vi "SRQ Event Handling.vi"() -> ()   [LabVIEW 2020]
doc: "This example detects and responds to a service request (SRQ) event. It shows a generic method to generate and handle an SRQ event. But each instrument that supports SRQ event assertion will use a different set of commands than what is shown in this example. You will need to refer to the programmer reference manual for your particular instrument to determine the correct set of commands."
uses:
  <vilib>/Instr/_visa.llb/Select Event Type.ctl
panel:
  in  "Command":string="*ESE 0x01; *SRE 0x30; SOUR:FUNC SIN;*OPC;SENS:DATA?"
  out "status byte":u16
  out "Raw Data":string
  in  "VISA GPIB Resource":refnum<visa-resource-name>="GPIB0::3::INSTR"
  # "Overview: Detects and responds to a service request (SRQ) event sent by a GPIB device.\nRequirements: NI-488.2 and NI-VISA Drivers\nInstructions:\n1. Ensure the resource specified in the VISA GPIB Resource control is properly configured in Measurement & Automation Explorer.\n2. Run the VI.\n3. If your instrument recognizes the Command specified below, it should return a response in the Raw Data."
  # "Service Request (SRQ) events are sent by GPIB devices to the controller to request service. The Command string in this example which instructs the instrument to generate an SRQ may need to be modified for your specific instrument."
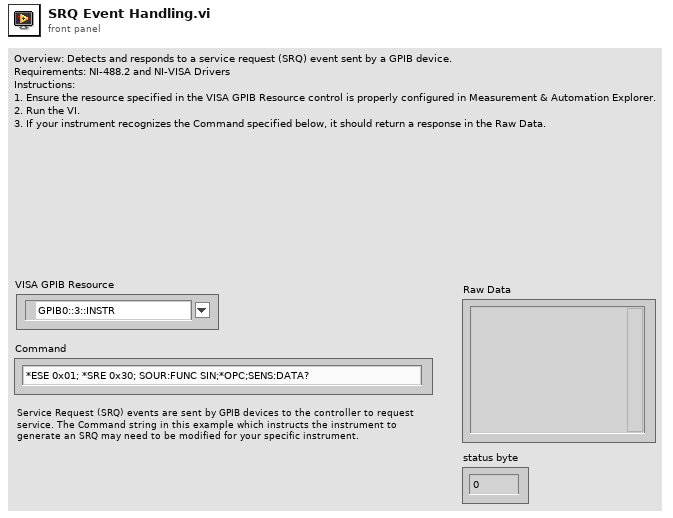
[diagram p1: front panel]
types:
  T1 = typedef "Select Event Type.ctl" = u32
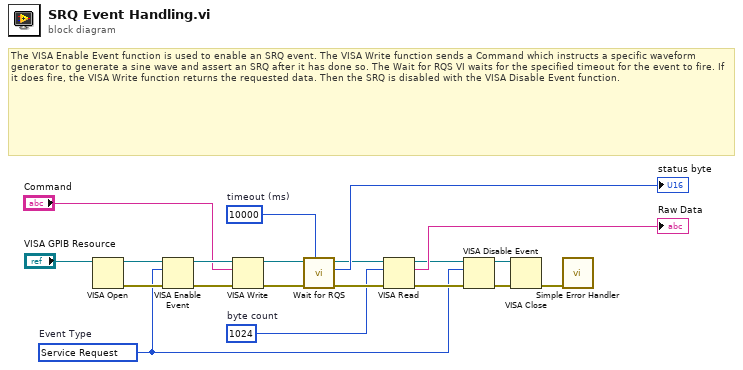
[diagram p0: block diagram]
diagram:
  w2 = u32 1024  # byte count
  w1 = u32 10000  # timeout (ms)
  w3 = T1 1073684491 items=["Service Request"=1073684491, "Trigger"=3221168138, "Clear"=1073684493, "VXI Signal"=1073684512, "VXI/VME Interrupt"=3221168161, "VXI/VME Sysfail"=1073684509, "VXI/VME Sysreset"=1073684510, "GPIB CIC"=1073684498, "GPIB Talk"=1073684499, "GPIB Listen"=1073684500, "PXI Interrupt"=1073684514, "Serial Break"=1073684515, "Serial TermChar"=1073684516, "Serial CTS"=1073684521, "Serial DSR"=1073684522, "Serial DCD"=1073684524, "Serial RI"=1073684526, "Serial Character"=1073684533, "USB Interrupt"=1073684535, "All Enabled"=1073709055]  # Event Type
  # "The VISA Enable Event function is used to enable an SRQ event. The VISA Write function sends a Command which instructs a specific waveform generator to generate a sine wave and assert an SRQ after it has done so. The Wait for RQS VI waits for the specified timeout for the event to fire. If it does fire, the VISA Write function returns the requested data. Then the SRQ is disabled with the VISA Disable Event function."
  n1 = VISA Open(VISA resource name="VISA GPIB Resource") -> (VISA resource name=w16:refnum<visa-resource-name>, error out=w17:errorcluster)  [unwired: 1 in, 3 out]
  n2 = VISA Enable Event(8:w17, 10:w3, 11:w16) -> (0:w18:errorcluster, 3:w15:refnum<visa-resource-name>)  [unwired: 1 out]
  n3 = VISA Write(VISA resource name=w15, write buffer="Command", error in (no error)=w18) -> (VISA resource name out=w14:refnum<visa-resource-name>, error out=w19:errorcluster)  [unwired: 1 out]
  n4 = call <vilib>:"Wait for RQS.VI"("timeout (25000 ms)"=w1, "error in (no error)"=w19, "VISA resource name"=w14) -> ("error out"=w4:errorcluster, "status byte"=→"status byte":u16, "VISA resource name out"=w5:refnum<visa-resource-name>)  [unwired: 2 in, 4 out]
  n5 = VISA Read(VISA resource name=w5, byte count=w2, error in (no error)=w4) -> (VISA resource name out=w10:refnum<visa-resource-name>, read buffer=→"Raw Data":string, error out=w8:errorcluster)  [unwired: 1 out]
  n6 = VISA Disable Event(8:w8, 10:w3, 11:w10) -> (0:w7:errorcluster, 3:w9:refnum<visa-resource-name>)  [unwired: 1 in]
  n7 = VISA Close(VISA resource name=w9, error in (no error)=w7) -> (error out=w11:errorcluster)
  n8 = call <vilib>:"Simple Error Handler.vi"("error in (no error)"=w11) -> ()  [unwired: 1 in, 8 out]
